vi "DriveTest.vi"() -> ()   [LabVIEW 2009]
uses:
  <vilib>/rvi/interface/nirviOpenFPGA/nirviOpenFPGA.xnode
  FPGA Bitfiles/scmproject.lvproj_FPGA Target_RobotFPGA.vi.lvbitx
  RobotFPGA.vi
  <vilib>/rvi/interface/RandomDataEmulation/nirviRandomDataOpen.vi
  <vilib>/rvi/interface/nirviOpenFPGA/nirviOpenFPGA.ctl
  <vilib>/rvi/interface/nirviOpenFPGA/nirviopenstate.ctl
  <vilib>/picture/picture.llb/imagedata.ctl
  <vilib>/rvi/interface/common/nirviIntfCommonState.ctl
  <vilib>/rvi/interface/common/nirviIntfModes.ctl
  C:/Program Files/National Instruments/LabVIEW 2009/resource/RVI/emulation/niLvFpgaEmulationMode.ctl
  <vilib>/eio/XNode/Errors/EIOXNodeErrorStruct.ctl
  <vilib>/eio/XNode/Errors/EIOXNodeInternalErrorTypes.ctl
  <vilib>/eio/XNode/Errors/EIOXNodeUserErrorTypes.ctl
  <vilib>/XNodeSupport/XNodeRect32.ctl
  <vilib>/XNodeSupport/XNodeInt.ctl
  <vilib>/XNodeSupport/XNodeTerms.ctl
  <vilib>/XNodeSupport/XNodeTerm.ctl
  <vilib>/XNodeSupport/XNodeString.ctl
  <vilib>/XNodeSupport/XNodeVariant.ctl
  <vilib>/XNodeSupport/XNodeBool.ctl
  <vilib>/rvi/interface/nirviCloseFPGA/nirviCloseFPGA.xnode
  <vilib>/rvi/interface/RandomDataEmulation/nirviRandomDataClose.vi
  Drive.lvlib
  <vilib>/userdefined/High Color/nirio_resource_hc.ctl
  <vilib>/XNodeSupport/NI_XNodeSupport.lvlib
panel:
  in  "stop":bool
  in  "Y_Speed":dbl(slide) min=-1.0 max=1.0 scale=-1.0..1.0
  in  "X_Speed":dbl(slide) min=-1.0 max=1.0 scale=-1.0..1.0
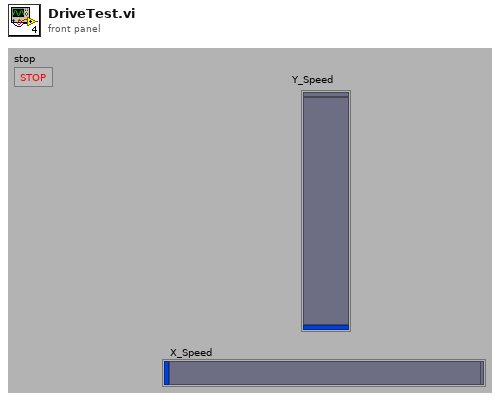
[diagram p1: front panel]
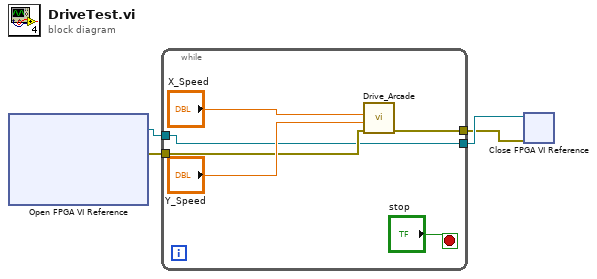
[diagram p0: block diagram]
diagram:
  n1 = xnode "Open FPGA VI Reference"() -> ("FPGA VI Reference Out"=w3:refnum<k20>, "error out"=w4:errorcluster)  [unwired: 2 in]
  n2 = while {
    tunnel: w4 -> [w7]
    tunnel: [w6] -> w1
    tunnel: w3 -> [w5]
    tunnel: [w5] -> w2
    stop <- "stop" stop-if-true
    n3 = call "Drive_Arcade.vi"("error in"=w7, "Y_Speed"="Y_Speed", "X_Speed"="X_Speed") -> ("error out"=w6:errorcluster)  [unwired: 8 in]
  }
  n4 = xnode "Close FPGA VI Reference"("FPGA VI Reference In"=w2, "error in"=w1) -> ()  [unwired: 1 out]
